vi "Add WebSocket Server.vi"(8 "error in (no error)":errorcluster, 9 "Request Path Regex (All)":string, 10 "WebSocket Server":refnum<class "Websocket Server.lvclass">, 11 "Server in":refnum<class "Server.lvclass">) -> (0 "error out":errorcluster, 3 "Server out":refnum<class "Server.lvclass">)   [LabVIEW 2020, in "HTTP Server.lvlib" / "Server.lvclass"]
uses:
  Server.lvclass
  lv-stream-websocket/Stream-Websocket/Websocket Server/Websocket Server.lvclass
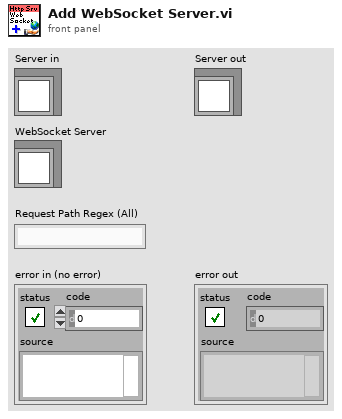
[diagram p1: front panel]
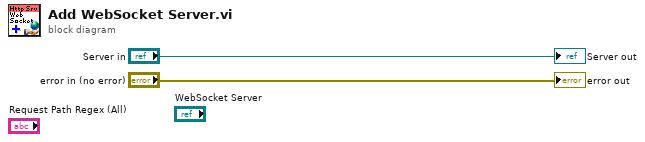
[diagram p0: block diagram]
diagram:
  "error out" <- "error in (no error)"
  "Server out" <- "Server in"
